vi "Planner_Screen.vi"(8 "error in (no error)":errorcluster) -> (0 "error out":errorcluster)   [LabVIEW 2017]
uses:
  Controls/Recipe_selection_loop.ctl
  Controls/cluster.ctl
  <vilib>/addons/database/Connection.llb/Conn ObjectReference.ctl
  <vilib>/Utility/error.llb/DialogType.ctl
  <vilib>/addons/database/Connection.llb/DB Tools Open Connec (Path).vi
  <vilib>/ethernetip/ethernetip.llb/EthernetIP SLC500 Write Integer.vi
  <vilib>/Utility/file.llb/Write Delimited Spreadsheet (string).vi
  <vilib>/addons/database/NI_Database_API.lvlib
  <vilib>/ethernetip/ethernetip.lvlib
panel:
  out "Quantity day":i32[](array[numeric])
  out "Recipe Names INDEX":i32[](array[numeric])
  out "TIME DATA":i32[](array[numeric])
  out "PLC upload DATA":i32[](array[numeric])
  out "data 2":string
  out "appended path 2":path
  out "Product List":string[][](array[string])
  out "data":string
  out "CtlRef":refnum<vi>
  out "Data DOWNLOAD":i16[][](array[numeric])
  out "STATION NUMBER":string[](array[string])
  out "MACHINE NAME":string[](array[string])
  out "IP Address":string[](array[string])
  in  "Home Square":bool
  in  "Tab Control":T1(tab)
  in  "Machine 1":T2 {"PLAN 4" format="%<%X\n%x>T"; "PLAN 3" format="%<%X\n%x>T"; "PLAN 2" format="%<%X\n%x>T"; "PLAN 1" format="%<%X\n%x>T"}
  in  "Machine 2":T3 caption="Machine 1" {"PLAN 4" format="%<%X\n%x>T"; "PLAN 3" format="%<%X\n%x>T"; "PLAN 2" format="%<%X\n%x>T"; "PLAN 1" format="%<%X\n%x>T"}
  in  "Machine 3":T3 caption="Machine 1" {"PLAN 4" format="%<%X\n%x>T"; "PLAN 3" format="%<%X\n%x>T"; "PLAN 2" format="%<%X\n%x>T"; "PLAN 1" format="%<%X\n%x>T"}
  in  "Machine 4":T3 caption="Machine 1" {"PLAN 4" format="%<%X\n%x>T"; "PLAN 3" format="%<%X\n%x>T"; "PLAN 2" format="%<%X\n%x>T"; "PLAN 1" format="%<%X\n%x>T"}
  in  "Machine 5":T3 caption="Machine 1" {"PLAN 4" format="%<%X\n%x>T"; "PLAN 3" format="%<%X\n%x>T"; "PLAN 2" format="%<%X\n%x>T"; "PLAN 1" format="%<%X\n%x>T"}
  in  "Machine 6":T3 caption="Machine 1" {"PLAN 4" format="%<%X\n%x>T"; "PLAN 3" format="%<%X\n%x>T"; "PLAN 2" format="%<%X\n%x>T"; "PLAN 1" format="%<%X\n%x>T"}
  in  "Machine 7":T3 caption="Machine 1" {"PLAN 4" format="%<%X\n%x>T"; "PLAN 3" format="%<%X\n%x>T"; "PLAN 2" format="%<%X\n%x>T"; "PLAN 1" format="%<%X\n%x>T"}
  in  "Machine 8":T3 caption="Machine 1" {"PLAN 4" format="%<%X\n%x>T"; "PLAN 3" format="%<%X\n%x>T"; "PLAN 2" format="%<%X\n%x>T"; "PLAN 1" format="%<%X\n%x>T"}
  in  "Machine 9":T3 caption="Machine 1" {"PLAN 4" format="%<%X\n%x>T"; "PLAN 3" format="%<%X\n%x>T"; "PLAN 2" format="%<%X\n%x>T"; "PLAN 1" format="%<%X\n%x>T"}
  in  "Machine 10":T3 caption="Machine 1" {"PLAN 4" format="%<%X\n%x>T"; "PLAN 3" format="%<%X\n%x>T"; "PLAN 2" format="%<%X\n%x>T"; "PLAN 1" format="%<%X\n%x>T"}
  out "String Indicator":string
  # "PRODUCTION PLANING  SELECTOR"
  # "DAY, MONTYH, YEAR, HOURS, MINUTE, RECIPE NAME, PRODUCT COUNT"
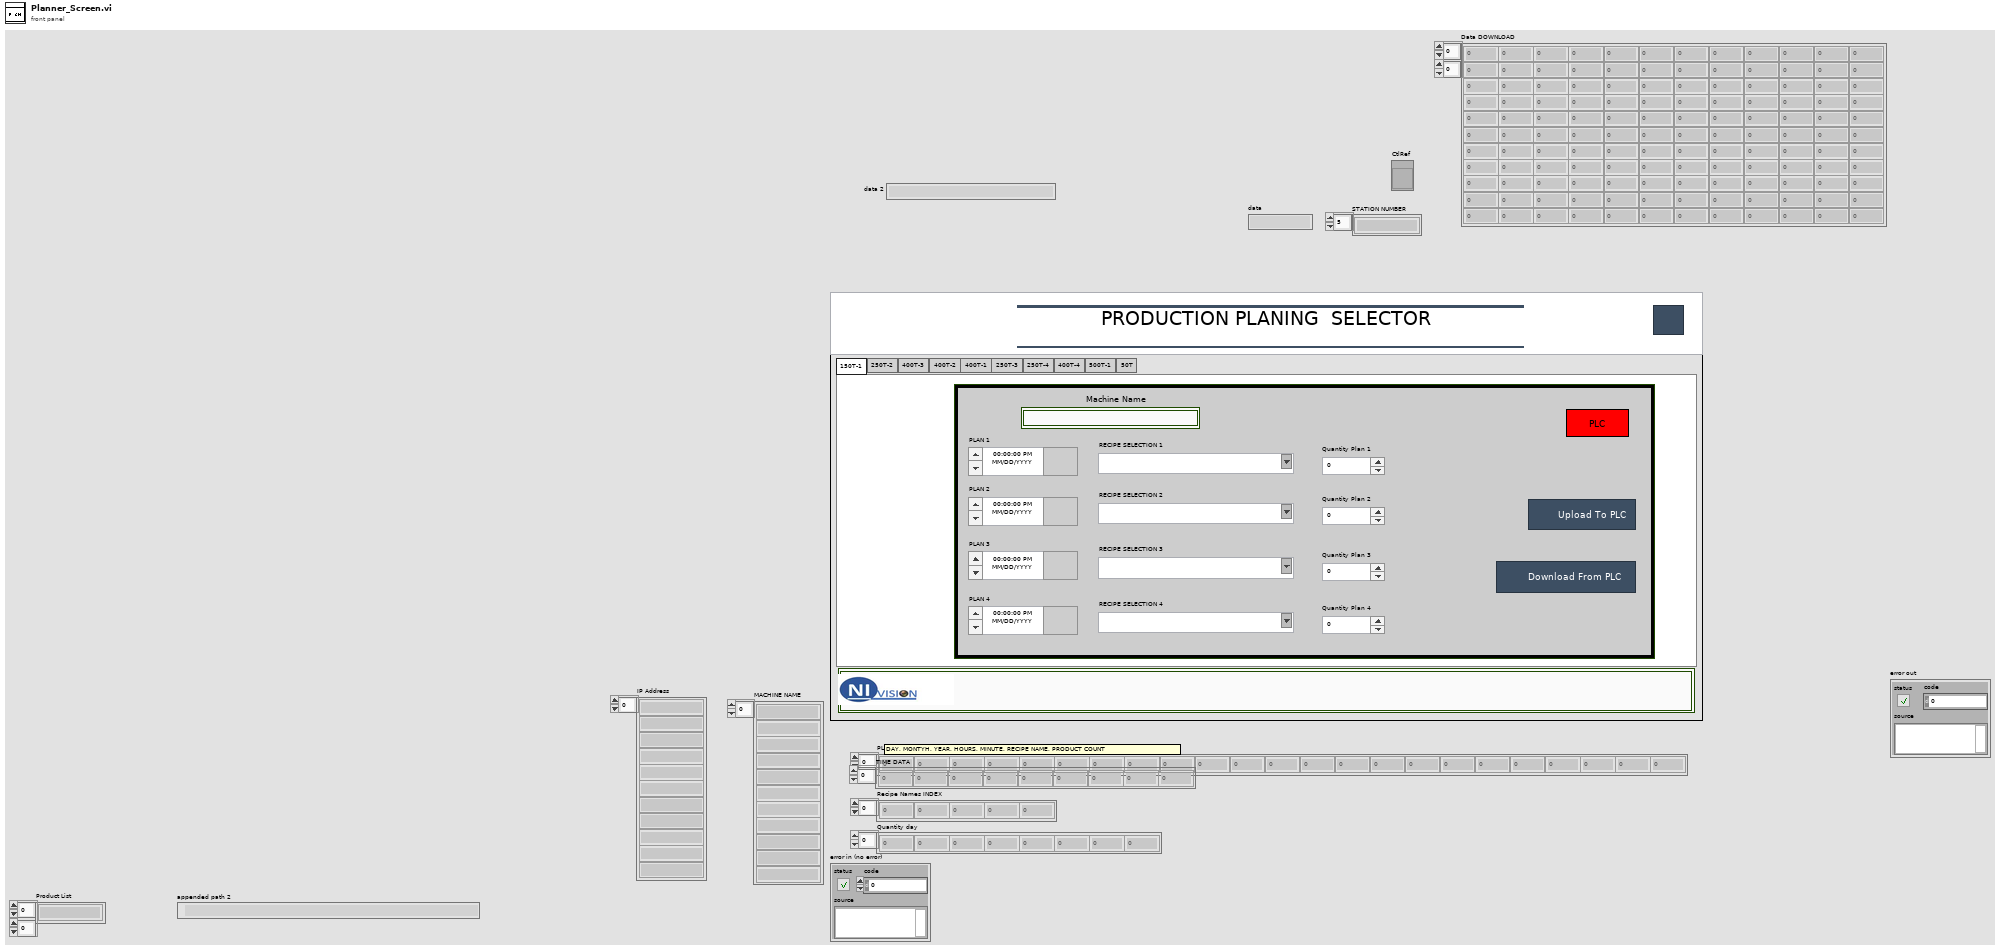
[diagram p1: front panel]
types:
  T1 = enum32{"MACHINE 1", "MACHINE 3", "MACHINE 4", "MACHINE 5", "MACHINE 6", "MACHINE 7", "MACHINE 8", "MACHINE 9", "MACHINE 10", "MACHINE 11"}
  T2 = cluster{"Machine Name":string, "Machine IP address":string, "PLAN 1 ":timestamp, "RECIPE SELECTION 1":string, "Download from PLC":bool, "Upload Button":bool, "PLC ":bool, "PLAN 2":timestamp, "RECIPE SELECTION 2":string, "PLAN 3":timestamp, "RECIPE SELECTION 3":string, "PLAN 4":timestamp, "RECIPE SELECTION 4":string, "Quantity Plan 1":i32, "Quantity Plan 2":i32, "Quantity Plan 3":i32, "Quantity Plan 4":i32, "TIME DATA":i32[]}
  T3 = cluster{"Machine Name":string, "Machine IP address":string, "PLAN 1 ":timestamp, "RECIPE SELECTION PLAN 1":string, "Download from PLC":bool, "Upload Button":bool, "PLC ":bool, "PLAN 2":timestamp, "RECIPE SELECTION PLAN 2":string, "PLAN 3":timestamp, "RECIPE SELECTION PLAN 3":string, "PLAN 4":timestamp, "RECIPE SELECTION PLAN 4":string, "Quantity Plan 1":i32, "Quantity Plan 2":i32, "Quantity Plan 3":i32, "Quantity Plan 4":i32}
  T4 = typedef "cluster.ctl" = cluster{"IP Address":string[], "Machine name":string[], "Station number":string[], "Product List":string[][], "Recipe_upload_history path":path, "reference":T5, "appended array":refnum<vi>[]}
  T5 = typedef "NI_Database_API.lvlib/Conn ObjectReference.ctl" = refnum<k1>
  T6 = typedef "Recipe_selection_loop.ctl" = enum16{"Init", "Init_2", "Start", "Upload_to_PLC", "Download_to_PLC", "Stop"}
  T7 = enum32{"invalid app kind", "Development System", "Run Time System", "Student Edition", "Embedded LabVIEW", "Evaluation", "Custom"}
  T8 = typedef "DialogType.ctl" = u16
  T9 = typedef "ethernetip.lvlib/ethernetip.ctl" = refnum<k21>
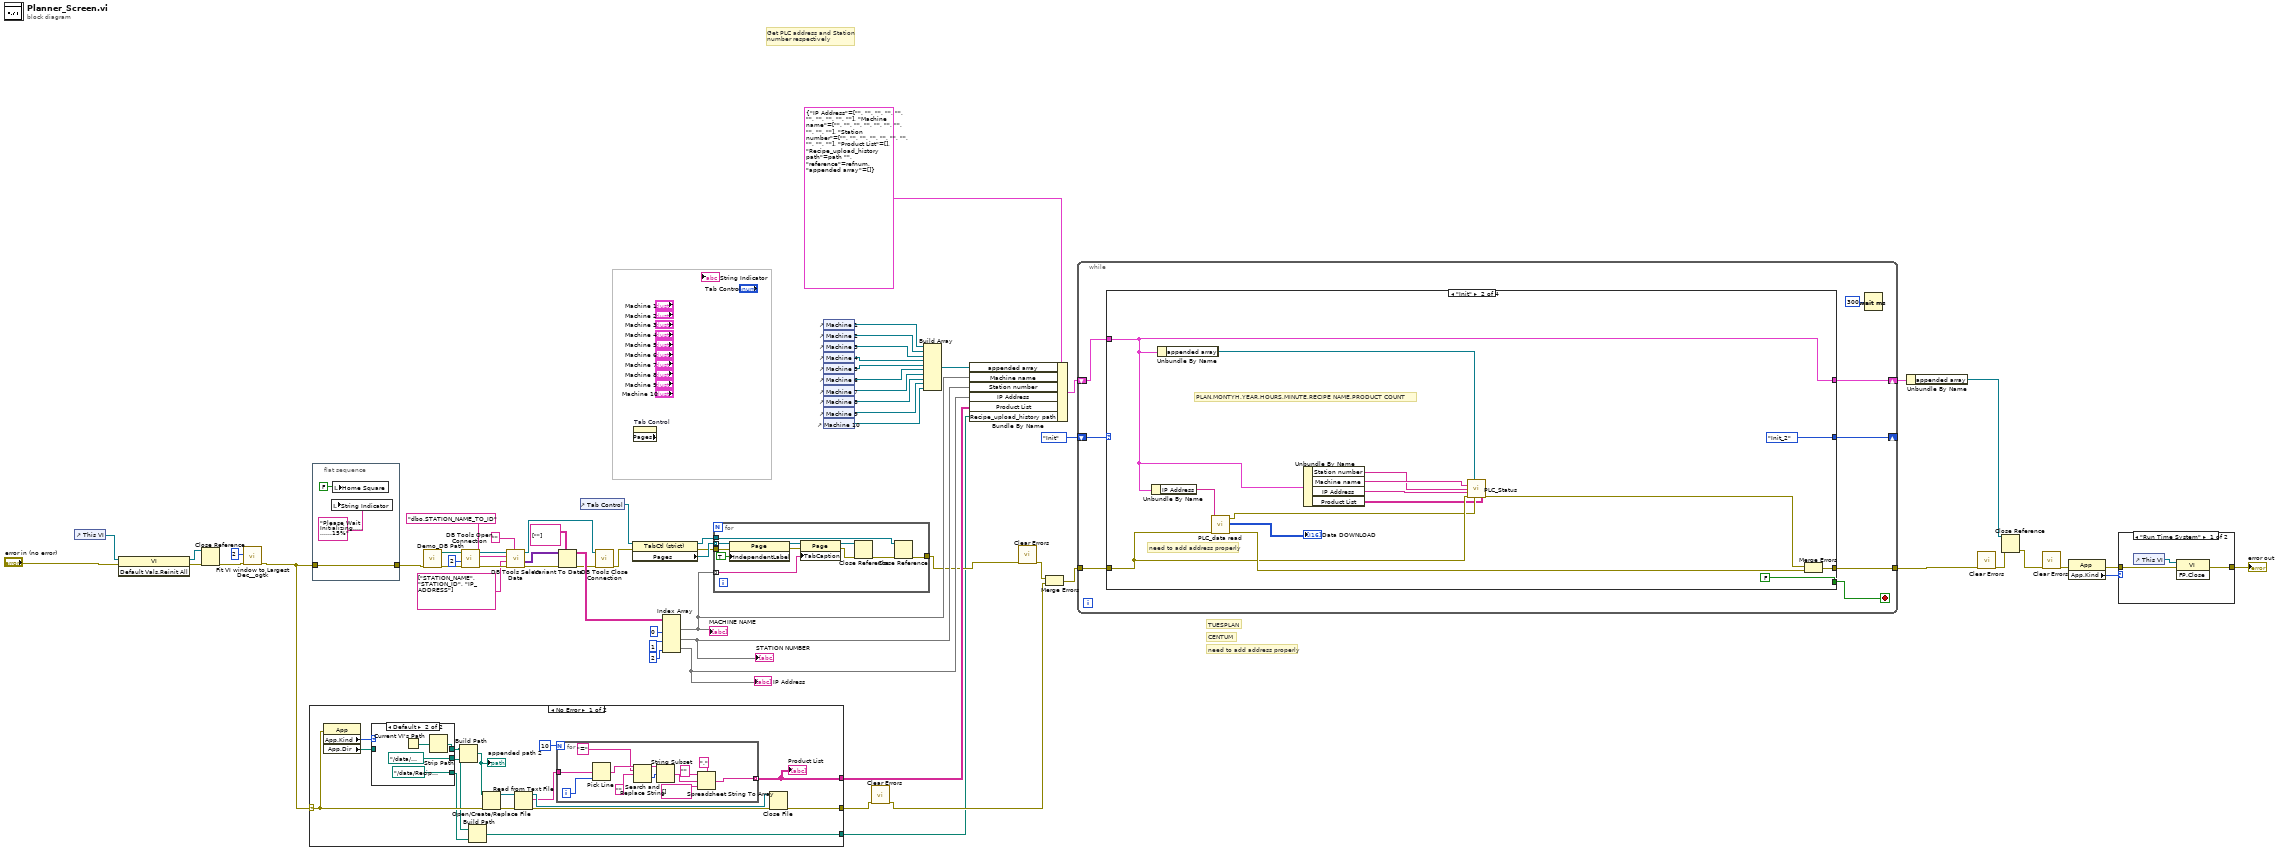
[diagram p0: block diagram]
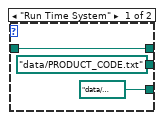
[diagram p3: hidden frame]
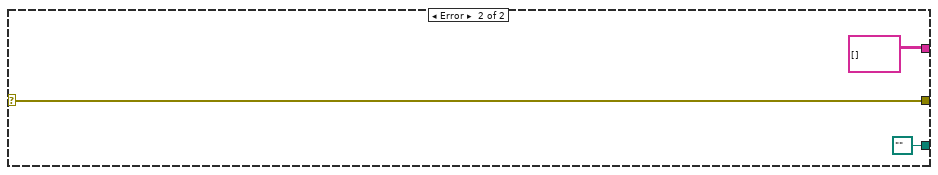
[diagram p4: hidden frame]
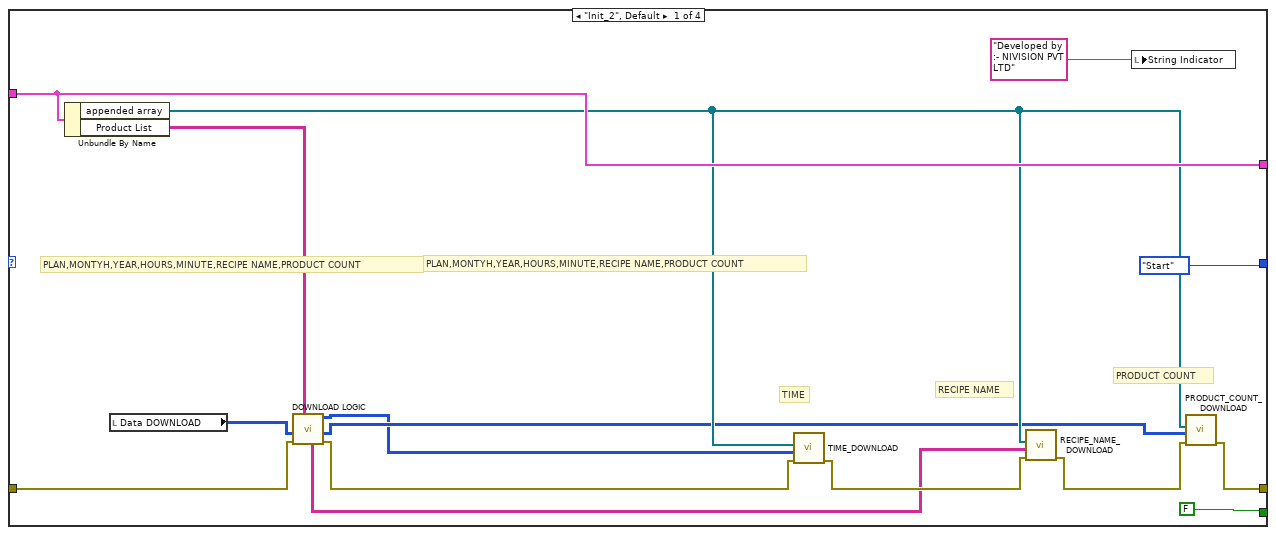
[diagram p5: hidden frame]
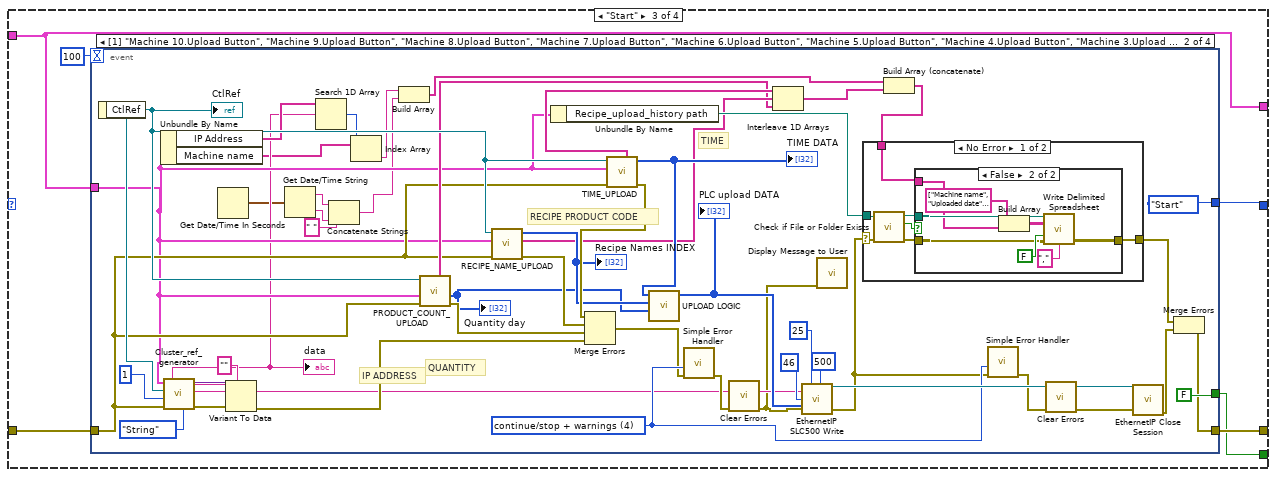
[diagram p6: hidden frame]
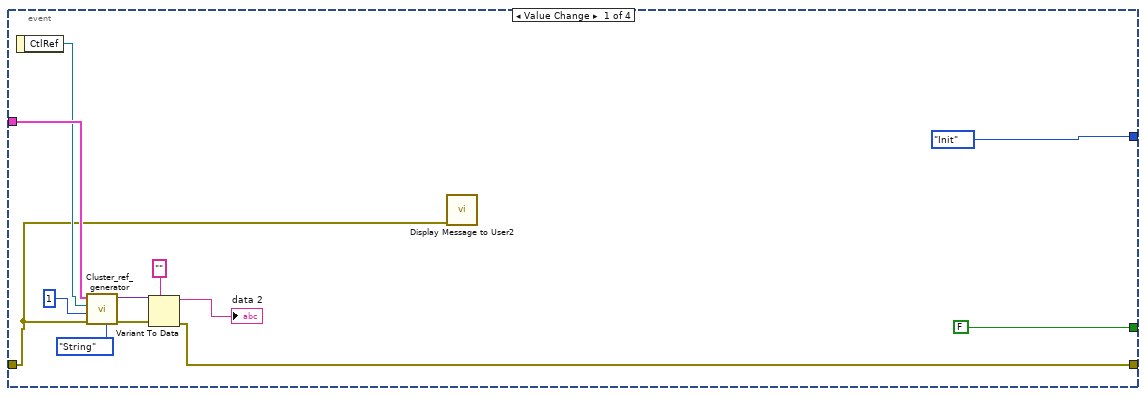
[diagram p7: hidden frame]
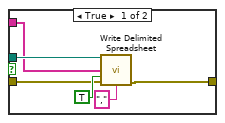
[diagram p8: hidden frame]
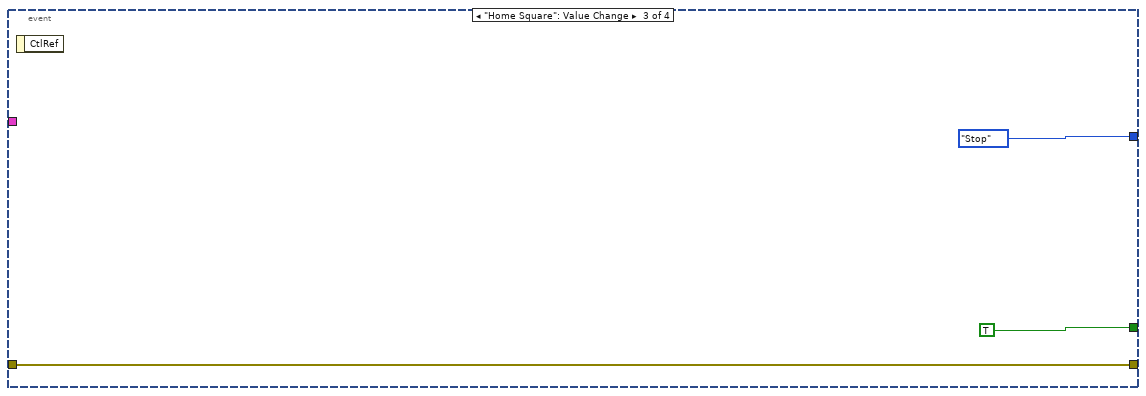
[diagram p10: hidden frame]
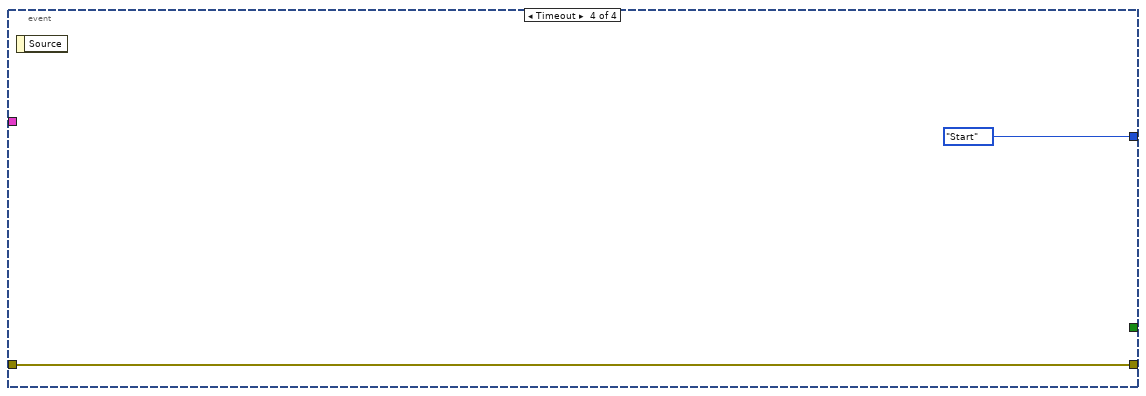
[diagram p11: hidden frame]
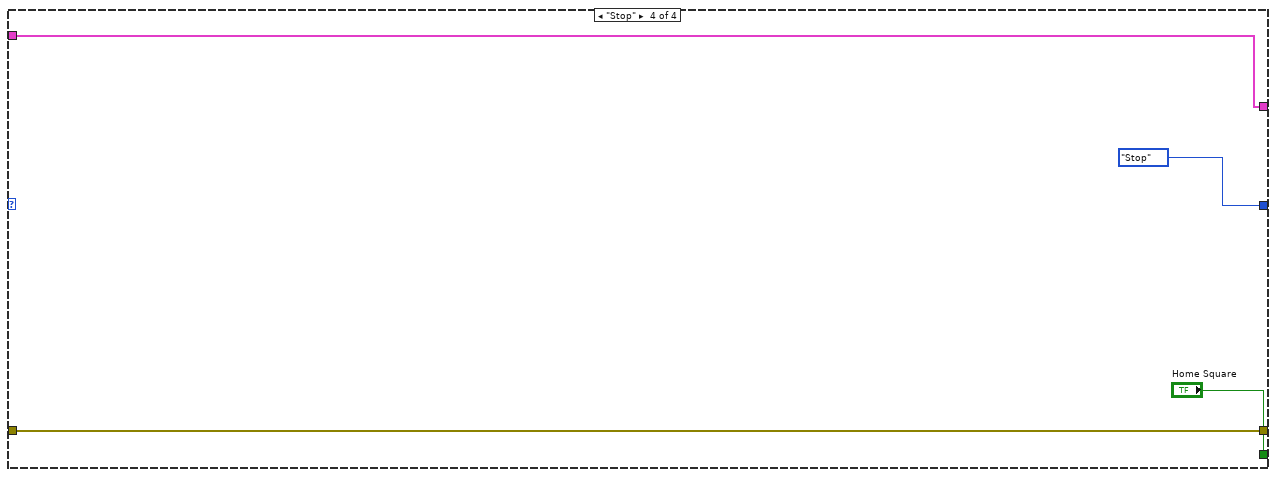
[diagram p12: hidden frame]
diagram:
  # "need to add address properly"
  # "CENTUM"
  # "TUESPLAN"
  # "Get PLC address and Station\nnumber respectively"
  n1 = control-ref of="This VI"() -> (w63:refnum<vi>)
  n2 = invoke class="VI" method="Default Vals.Reinit All"(reference=w63, error in="error in (no error)") -> (reference out=w62:refnum<vi>, error out=w61:errorcluster)  [unwired: 1 in, 1 out]
  n3 = Close Reference(reference=w62, error in (no error)=w61) -> (error out=w9:errorcluster)
  n4 = call <userlib>:"Fit VI window to Largest Dec__ogtk.vi"("error in (no error)"=w9, "border spacing (2 px)"=2) -> ("error out"=w8:errorcluster)  [unwired: 4 in, 1 out]
  n5 = case shown="No Error" w8 {
    selector: w8 -> [w68 w101]
    tunnel: [w71 w101] -> w13
    tunnel: [w67 string[][] [] ("delimiter (Tab)")] -> w14
    tunnel: [w64 path "" ("appended path")] -> w1
    frame No Error {
      n6 = property class="App"(error in=w68) -> ("App.Kind"=w79:T7, "App.Dir"=w78:path)  [unwired: 1 in, 2 out]
      n7 = case shown="Default" w79 {
        tunnel: w78 -> [w94 _]
        tunnel: [path "data/PRODUCT_CODE.txt" ("path") path "../data/PRODUCT_CODE.txt" ("path")] -> w76
        tunnel: [w94 w96] -> w66
        tunnel: [path "data/Recipe_Uploaded_History.csv" ("path") path "../data/Recipe_Uploaded_History.csv" ("path")] -> w65
        frame "Run Time System" {
        }
        frame Default {
          n8 = Current VI's Path() -> (path=w97:path)
          n9 = Strip Path(path=w97) -> (stripped path=w96:path)  [unwired: 1 out]
        }
      }
      n10 = Build Path(base path=w66, name or relative path=w76) -> (appended path=w77:path)
      "appended path 2" <- w77
      n11 = Build Path(base path=w66, name or relative path=w65) -> (appended path=w64:path)
      n12 = Open/Create/Replace File(file path (use dialog)=w77, error in=w68) -> (refnum out=w75:refnum<file>, error out=w74:errorcluster)  [unwired: 4 in, 1 out]
      n13 = Read from Text File(file (use dialog)=w75, error in=w74) -> (refnum out=w72:refnum<file>, text=w70:string, error out=w73:errorcluster)  [unwired: 2 in, 1 out]
      n14 = for {
        N: 10 -> [_]
        tunnel: w70 -> [w82]
        tunnel: [w80] -> w67 mode=indexing
        i -> [w83]
        n15 = Pick Line(multi-line string=w82, line index=w83) -> (output string=w84:string)  [unwired: 1 in]
        n16 = Search and Replace String(input string=w84, search string="=" ("format string"), replace string="" ("search string")) -> (result string=w86:string, offset past replacement=w87:i32)  [unwired: 5 in, 2 out]
        n17 = String Subset(string=w86, offset (0)=w87) -> (substring=w85:string)  [unwired: 1 in]
        n18 = Spreadsheet String To Array(delimiter (Tab)=",", format string="", spreadsheet string=w85, array type (2D Dbl)=string[] [] ("delimiter (Tab)")) -> (array=w80:string[])
      }
      "Product List" <- w67
      n19 = Close File(refnum=w72, error in=w73) -> (error out=w71:errorcluster)  [unwired: 1 out]
    }
    frame Error {
    }
  }
  n20 = flat-sequence {
    tunnel: [w104] -> w41
    tunnel: w8 -> [w104]
    frame #0 {
      n21 = local write "String Indicator"("Please Wait Initializing...........15%" ("String")) -> ()
      n22 = local write "Home Square"(FALSE) -> ()
    }
  }
  n23 = call "Demo_DB Path.vi"("error in"=w41) -> ("error out"=w57:errorcluster, "DB Path"=w58:path)  [unwired: 9 in]
  n24 = call-poly <vilib>:"DB Tools Open Connection.vi"("error in (no error)"=w57, "connection timeout (15)"=2, "connection information"=w58) -> ("error out"=w60:errorcluster, "connection reference"=w59:T5)  [unwired: 5 in]
  n25 = call <vilib>:"DB Tools Select Data.vi"("condition"="", "error in (no error)"=w60, "columns"=string[] ["STATION_NAME", "STATION_ID", "IP_ADDRESS"], "table"="dbo.STATION_NAME_TO_ID", "connection reference"=w59) -> ("error out"=w49:errorcluster, "data"=w50:variant[][], "connection reference out"=w20:T5)  [unwired: 1 in]
  n26 = Variant To Data(error in=w49, type=string[][] [[""]], Variant=w50) -> (data=w45:string[][], error out=w19:errorcluster)
  n27 = control-ref of="Tab Control"() -> (w44:refnum<vi>)
  n28 = call <vilib>:"DB Tools Close Connection.vi"("error in (no error)"=w19, "connection reference"=w20) -> ("error out"=w18:errorcluster)  [unwired: 5 in]
  n29 = property class="TabCtl (strict)"(reference=w44, error in=w18) -> (reference out=w27:refnum<vi>, error out=w42:errorcluster, "Pages"=w43:refnum<vi>[])
  n30 = property on="Tab Control" class="TabCtl (strict)" props=["Pages"]() -> ()  [unwired: 2 in, 3 out]
  n31 = Index Array(array=w45, index (col) #1=0 ("disabled index (col)"), index (col) #2=1 ("disabled index (col)"), index (col) #3=2 ("disabled index (col)")) -> (element #1=w37:string[], element #2=w15:string[], element #3=w16:string[])  [unwired: 3 in]
  "IP Address" <- w16
  "MACHINE NAME" <- w37
  "STATION NUMBER" <- w15
  n32 = for {
    tunnel: w43 -> [w115] mode=indexing
    tunnel: w42 -> [w113]
    tunnel: [w106] -> w11
    tunnel: w37 -> [w108] mode=indexing
    tunnel: w27 -> [w105]
    n33 = property class="Page"(reference=w115, error in=w113, "IndependentLabel"=TRUE) -> (reference out=w112:refnum<vi>, error out=w109:errorcluster)
    n34 = property class="Page"(reference=w112, error in=w109, "TabCaption"=w108) -> (reference out=w111:refnum<vi>, error out=w110:errorcluster)
    n35 = Close Reference(reference=w111, error in (no error)=w110) -> (error out=w107:errorcluster)
    n36 = Close Reference(reference=w105, error in (no error)=w107) -> (error out=w106:errorcluster)
  }
  n37 = control-ref of="Machine 1"() -> (w26:refnum<vi>)
  n38 = control-ref of="Machine 2"() -> (w36:refnum<vi>)
  n39 = control-ref of="Machine 3"() -> (w35:refnum<vi>)
  n40 = control-ref of="Machine 4"() -> (w34:refnum<vi>)
  n41 = control-ref of="Machine 5"() -> (w33:refnum<vi>)
  n42 = control-ref of="Machine 6"() -> (w32:refnum<vi>)
  n43 = control-ref of="Machine 7"() -> (w31:refnum<vi>)
  n44 = control-ref of="Machine 8"() -> (w30:refnum<vi>)
  n45 = control-ref of="Machine 9"() -> (w29:refnum<vi>)
  n46 = control-ref of="Machine 10"() -> (w28:refnum<vi>)
  n47 = call <vilib>:"Clear Errors.vi"("error in (no error)"=w13) -> ("error out"=w12:errorcluster)  [unwired: 5 in, 1 out]
  n48 = Build Array(w26, w36, w35, w34, w33, w32, w31, w30, w29, w28) -> (w25:refnum<vi>[])
  n49 = Bundle By Name(cluster=T4 {"IP Address"=["", "", "", "", "", "", "", "", "", ""], "Machine name"=["", "", "", "", "", "", "", "", "", ""], "Station number"=["", "", "", "", "", "", "", "", "", ""], "Product List"=[], "Recipe_upload_history path"=path "", "reference"=refnum, "appended array"=[]}, "appended array"=w25, "Machine name"=w37, "Station number"=w15, "IP Address"=w16, "Product List"=w14, "Recipe_upload_history path"=w1) -> (w39:T4)
  n50 = call <vilib>:"Clear Errors.vi"("error in (no error)"=w11) -> ("error out"=w10:errorcluster)  [unwired: 5 in, 1 out]
  n51 = Merge Errors(w10, w12) -> (w17:errorcluster)
  n52 = while {
    tunnel: w17 -> [w122]
    shift-right: [w120] -> w22
    shift-left: w39 -> [w119]
    tunnel: [w118] -> w23
    shift-right: [w117] -> _
    shift-left: Recipe_selection_loop."Init" ("Enum") -> [w121]
    stop <- w116 stop-if-true
    n53 = case shown="\"Init\"" w121 {
      tunnel: w122 -> [w131 w142 w155 w250]
      tunnel: [w134 w152 w159 w250] -> w118
      tunnel: [w136 w143 w154 w251] -> w120
      tunnel: w119 -> [w136 w143 w154 w251]
      tunnel: [Recipe_selection_loop."Start" ("Enum") Recipe_selection_loop."Init_2" ("Enum") w157 Recipe_selection_loop."Stop" ("Enum")] -> w117
      tunnel: [FALSE FALSE w156 "Home Square"] -> w116
      frame "Init_2", Default {
        # "PLAN,MONTYH,YEAR,HOURS,MINUTE,RECIPE NAME,PRODUCT COUNT"
        # "TIME"
        # "PRODUCT COUNT"
        # "RECIPE NAME"
        # "PLAN,MONTYH,YEAR,HOURS,MINUTE,RECIPE NAME,PRODUCT COUNT"
        n54 = Unbundle By Name(w136) -> ("appended array"=w132:refnum<vi>[], "Product List"=w127:string[][])
        n55 = local read "Data DOWNLOAD"() -> (w129:i16[][])
        n56 = call "DOWNLOAD LOGIC.vi"("Product List"=w127, "error in (no error)"=w131, "DATA"=w129) -> ("error out"=w130:errorcluster, "product count"=w128:i32[][], "DAy,month,year,hours,minute"=w125:i64[][], "recipe names"=w126:string[][])  [unwired: 4 in, 1 out]
        n57 = call "TIME_DOWNLOAD.vi"("error in (no error)"=w130, "Year,Month,Day,hour,Minute"=w125, "appended array"=w132) -> ("error out"=w133:errorcluster)  [unwired: 8 in]
        n58 = call "RECIPE_NAME_DOWNLOAD.vi"("error in (no error)"=w133, "Recipe Names"=w126, "appended array"=w132) -> ("error out"=w135:errorcluster)  [unwired: 8 in]
        n59 = local write "String Indicator"("Developed by :- NIVISION PVT LTD" ("String")) -> ()
        n60 = call "PRODUCT_COUNT_DOWNLOAD.vi"("error in (no error)"=w135, "Quantity Day"=w128, "appended array"=w132) -> ("error out"=w134:errorcluster)  [unwired: 8 in]
      }
      frame "Init" {
        # "PLAN,MONTYH,YEAR,HOURS,MINUTE,RECIPE NAME,PRODUCT COUNT"
        # "need to add address properly"
        n61 = Unbundle By Name(w143) -> ("IP Address"=w145:string[])
        n62 = Unbundle By Name(w143) -> ("appended array"=w153:refnum<vi>[])
        n63 = call "PLC_data read.vi"("error in (no error)"=w142, "IP Address"=w145) -> ("error out"=w151:errorcluster, "Data"=→"Data DOWNLOAD":i16[][], "Array"=w141:errorcluster[])  [unwired: 7 in]
        n64 = Unbundle By Name(w143) -> ("Station number"=w140:string[], "Machine name"=w146:string[], "IP Address"=w144:string[], "Product List"=w139:string[][])
        n65 = call "PLC_Status.vi"("appended array"=w153, "Machine name"=w146, "Station number"=w140, "IP Address"=w144, "error in (no error)"=w142, "PLC Status"=w141, "Recipe Names"=w139) -> ("error out"=w150:errorcluster)  [unwired: 8 in]
        n66 = Merge Errors(w150, w151) -> (w152:errorcluster)
      }
      frame "Start" {
        n67 = event shown="[1] \"Machine 10.Upload Button\", \"Machine 9.Upload Button\", \"Machine 8.Upload Button\", \"Machine 7.Upload Button\", \"Machine 6.Upload Button\", \"Machine 5.Upload Button\", \"Machine 4.Upload Button\", \"Machine 3.Upload Button\", \"Machine 2.Upload Button\", \"Machine 1.Upload Button\": Value Change" {
          selector: _ -> [_ _ _ _]
          dyn-events: _ -> [_ _ _ _]
          timeout: 100 -> [_ _ _ _]
          tunnel: [w162 w180 w244 w246] -> w159
          tunnel: w155 -> [w160 w189 w244 w246]
          tunnel: [Recipe_selection_loop."Init" ("Enum") Recipe_selection_loop."Start" ("Enum") Recipe_selection_loop."Stop" ("Enum") Recipe_selection_loop."Start" ("Enum")] -> w157
          tunnel: [FALSE FALSE TRUE _] -> w156
          tunnel: w154 -> [w164 w188 _ _]
          event "Machine 10.Download from PLC", "Machine 9.Download from PLC", "Machine 7.Download from PLC", "Machine 6.Download from PLC", "Machine 5.Download from PLC", "Machine 4.Download from PLC", "Machine 3.Download from PLC", "Machine 2.Download from PLC", "Machine 1.Download from PLC", "Machine 8.Download from PLC": Value Change {
            n68 = event-data() -> ("CtlRef"=w163:refnum<vi>)  [unwired: 1 in]
            n69 = call "Cluster_ref_generator.vi"("Cluster"=w164, "CtlRef"=w163, "Index from Cluster"=1, "error in (no error)"=w160, "Type"=enum16{"String", "Numeric", "Boolean", ""}."String") -> ("Value"=w166:variant, "error out"=w167:errorcluster)  [unwired: 4 in]
            n70 = Variant To Data(error in=w167, type="", Variant=w166) -> (data=→"data 2":string, error out=w162:errorcluster)
            n71 = call "Display Message to User2"("error in (no error)"=w160) -> ()  [unwired: 9 in, 2 out]
          }
          event "Machine 10.Upload Button", "Machine 9.Upload Button", "Machine 8.Upload Button", "Machine 7.Upload Button", "Machine 6.Upload Button", "Machine 5.Upload Button", "Machine 4.Upload Button", "Machine 3.Upload Button", "Machine 2.Upload Button", "Machine 1.Upload Button": Value Change {
            w198 = T8 4 items=["no dialog", "OK message", "continue or stop message", "OK message + warnings", "continue/stop + warnings"] ("type of dialog (OK msg:1)")
            # "IP ADDRESS"
            # "QUANTITY"
            # "RECIPE PRODUCT CODE"
            # "TIME"
            n72 = event-data() -> ("CtlRef"=w210:refnum<vi>)  [unwired: 1 in]
            "CtlRef" <- w210
            n73 = Unbundle By Name(w188) -> ("IP Address"=w187:string[], "Machine name"=w184:string[])
            n74 = call "Cluster_ref_generator.vi"("Cluster"=w188, "CtlRef"=w210, "Index from Cluster"=1, "error in (no error)"=w189, "Type"=enum16{"String", "Numeric", "Boolean", ""}."String") -> ("Value"=w215:variant, "error out"=w216:errorcluster)  [unwired: 4 in]
            n75 = Get Date/Time In Seconds() -> (seconds since 1Jan1904=w179:timestamp)
            n76 = Variant To Data(error in=w216, type="", Variant=w215) -> (data=w186:string, error out=w213:errorcluster)
            "data" <- w186
            n77 = Get Date/Time String(seconds (now)=w179) -> (date string=w175:string, time string=w176:string)  [unwired: 2 in]
            n78 = Search 1D Array(1D array=w187, element=w186) -> (index of element=w185:i32)  [unwired: 1 in]
            n79 = Concatenate Strings(w175, " " ("string"), w176) -> (w174:string)
            n80 = Index Array(array=w184, index=w185) -> (element=w178:string)
            n81 = Build Array(w178, w174) -> (w192:string[])
            n82 = call "PRODUCT_COUNT_UPLOAD.vi"("error in (no error)"=w189, "Cluster"=w188, "CtlRef"=w210) -> ("error out"=w211:errorcluster, "Quantity Day"=w205:i32[], "Quantity"=w193:string[])  [unwired: 6 in]
            "Quantity day" <- w205
            n83 = call "RECIPE_NAME_UPLOAD.vi"("CtlRef"=w210, "Cluster"=w188, "error in (no error)"=w189) -> ("Recipe Names INDEX"=w206:i32[], "Recipe Names"=w194:string[], "error out"=w212:errorcluster)  [unwired: 5 in]
            "Recipe Names INDEX" <- w206
            n84 = Unbundle By Name(w188) -> ("Recipe_upload_history path"=w196:path)
            n85 = call "TIME_UPLOAD.vi"("error in (no error)"=w189, "Cluster"=w188, "CtlRef"=w210) -> ("error out"=w209:errorcluster, "TIME DATA"=w207:i32[], "Time day"=w195:string[])  [unwired: 6 in]
            "TIME DATA" <- w207
            n86 = Merge Errors(w209, w212, w211, w213) -> (w183:errorcluster)
            n87 = call "UPLOAD LOGIC.vi"("Quantity day"=w205, "Recipe Names INDEX"=w206, "TIME DATA"=w207) -> ("PLC DATA"=w204:i32[])  [unwired: 8 in]
            "PLC upload DATA" <- w204
            n88 = call <vilib>:"Simple Error Handler.vi"("type of dialog (OK msg:1)"=w198, "error in (no error)"=w183) -> ("error out"=w208:errorcluster)  [unwired: 3 in, 4 out]
            n89 = call <vilib>:"Clear Errors.vi"("error in (no error)"=w208) -> ("error out"=w173:errorcluster)  [unwired: 5 in, 1 out]
            n90 = Interleave 1D Arrays(w195, w194, w193) -> (w191:string[])
            n91 = call-poly <vilib>:"EthernetIP SLC500 Write.vi"("File Number"=u16 25, "Timeout (ms)"=500, "Network Path"=w186, "Element Number"=u16 46, "Data"=w204, "error in"=w173) -> ("Session out"=w203:T9, "error out"=w172:errorcluster)  [unwired: 8 in]
            n92 = call "Display Message to User"("error in (no error)"=w173) -> ()  [unwired: 9 in, 2 out]
            n93 = Build Array (concatenate)(w192, w191) -> (w190:string[])
            n94 = case shown="No Error" w172 {
              selector: w172 -> [w224 w242]
              tunnel: [w227 w242] -> w182
              tunnel: w196 -> [w226 _]
              tunnel: w190 -> [w221 _]
              frame No Error {
                n95 = call <vilib>:"Check if File or Folder Exists.vi"("error in (no error)"=w224, "path"=w226) -> ("error out"=w223:errorcluster, "file or folder exists?"=w222:bool, "dup path"=w225:path)  [unwired: 7 in]
                n96 = case shown="False" w222 {
                  tunnel: [w233 w241] -> w227
                  tunnel: w225 -> [w230 w238]
                  tunnel: w223 -> [w229 w237]
                  tunnel: w221 -> [w228 w235]
                  frame True {
                    n97 = call-poly <vilib>:"Write Delimited Spreadsheet.vi"("file path (dialog if empty)"=w230, "1D data"=w228, "append to file? (new file:F)"=TRUE, "error in (no error)"=w229, "delimiter (\\t)"="," ("delimiter (\\t)")) -> ("error out"=w233:errorcluster)  [unwired: 9 in, 1 out]
                  }
                  frame False {
                    n98 = Build Array(string[] ["Machine name", "Uploaded date", "Plan 1 time", "Recipe 1 ", "Quantity 1", "Plan 2 time", "Recipe 2", "Quantity 2", "Plan 3 time", "Recipe 3", "Quantity 3", "Plan 4 time", "Recipe 4", "Quantity 5"] ("Array"), w235) -> (w236:string[][])
                    n99 = call-poly <vilib>:"Write Delimited Spreadsheet.vi"("file path (dialog if empty)"=w238, "2D data"=w236, "append to file? (new file:F)"=FALSE, "error in (no error)"=w237, "delimiter (\\t)"="," ("delimiter (\\t)")) -> ("error out"=w241:errorcluster)  [unwired: 9 in, 1 out]
                  }
                }
              }
              frame Error {
              }
            }
            n100 = call <vilib>:"Simple Error Handler.vi"("type of dialog (OK msg:1)"=w198, "error in (no error)"=w172) -> ("error out"=w197:errorcluster)  [unwired: 3 in, 4 out]
            n101 = call <vilib>:"Clear Errors.vi"("error in (no error)"=w197) -> ("error out"=w202:errorcluster)  [unwired: 5 in, 1 out]
            n102 = call <vilib>:"EthernetIP Close Session.vi"("error in"=w202, "Session in"=w203) -> ("error out"=w181:errorcluster)  [unwired: 9 in]
            n103 = Merge Errors(w182, w181) -> (w180:errorcluster)
          }
          event "Home Square": Value Change {
            n104 = event-data() -> ()  [unwired: 1 in, 1 out]
          }
          event Timeout {
            n105 = event-data() -> ()  [unwired: 1 in, 1 out]
          }
        }
      }
      frame "Stop" {
      }
    }
    n106 = Wait (ms)(milliseconds to wait=u32 300) -> ()  [unwired: 1 out]
  }
  n107 = Unbundle By Name(w22) -> ("appended array"=w21:refnum<vi>[])
  n108 = call <vilib>:"Clear Errors.vi"("error in (no error)"=w23) -> ("error out"=w24:errorcluster)  [unwired: 5 in, 1 out]
  n109 = Close Reference(reference=w21, error in (no error)=w24) -> (error out=w3:errorcluster)
  n110 = call <vilib>:"Clear Errors.vi"("error in (no error)"=w3) -> ("error out"=w4:errorcluster)  [unwired: 5 in, 1 out]
  n111 = property class="App"(error in=w4) -> (error out=w6:errorcluster, "App.Kind"=w5:T7)  [unwired: 1 in, 1 out]
  n112 = case shown="\"Run Time System\"" w5 {
    tunnel: [w252 w255] -> w2
    tunnel: w6 -> [w253 w255]
    frame "Run Time System" {
      n113 = control-ref of="This VI"() -> (w254:refnum<vi>)
      n114 = invoke class="VI" method="FP.Close"(reference=w254, error in=w253) -> (error out=w252:errorcluster)  [unwired: 1 in, 2 out]
    }
    frame "Development System", Default {
    }
  }
  "error out" <- w2
